vi "Delete Chan Group.vi"(8 "error in (no error)":errorcluster, 11 "Cfg Grandmaster in":refnum<class "Cfg Grandmaster.lvclass">) -> (0 "error out":errorcluster, 3 "Cfg Grandmaster out":refnum<class "Cfg Grandmaster.lvclass">)   [LabVIEW 2012, in "Configuration Grandmaster.lvlib" / "Cfg Grandmaster.lvclass"]
uses:
  Cfg Grandmaster.lvclass
  Cfg Grandmaster.lvclass/Cfg Grandmaster.ctl
  Class Chassis Cfg/ChassisCfg.lvclass
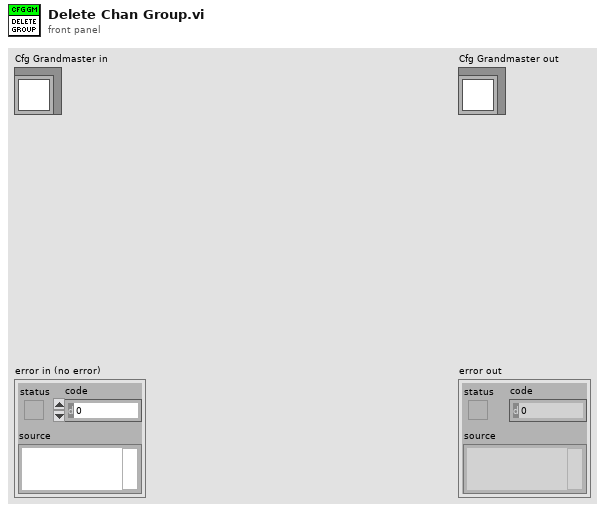
[diagram p1: front panel]
types:
  T1 = typedef "ge_Cfg wChassis.ctl" = cluster{"Chassis BOM":refnum<class "Chassis BOM.lvclass">, "Chassis Cfg":refnum<class "ChassisCfg.lvclass">, "Chassis Tasks":refnum<class "Chassis Tasks.lvclass">, "HW Error":bool, "Unsvd Chgs?":bool}
  T2 = typedef "Selected Group.ctl" = cluster{"ChanGroup":i32, "Rate Class":T3}
  T3 = typedef "TE_Designator.ctl" = enum16{"High Speed", "Low Speed"}
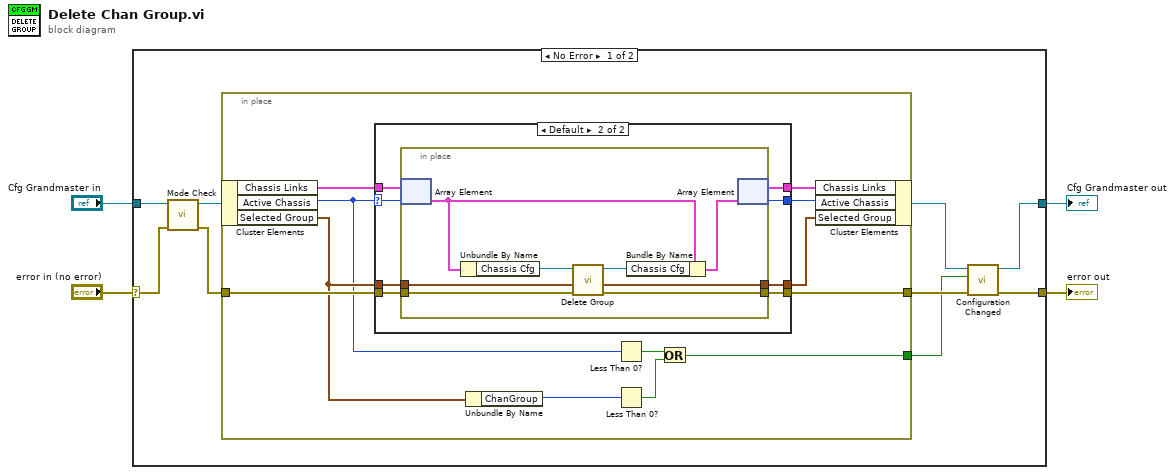
[diagram p0: block diagram]
diagram:
  n1 = case shown="No Error" "error in (no error)" {
    selector: "error in (no error)" -> [w10 w47]
    tunnel: [w8 w47] -> w3
    tunnel: [w6 w46] -> w1
    tunnel: "Cfg Grandmaster in" -> [w13 w46]
    frame No Error {
      n2 = call "Mode Check.vi"("error in (no error)"=w10, "Cfg Grandmaster in"=w13) -> ("error out"=w11:errorcluster, "Cfg Grandmaster out"=w12:refnum<class "Cfg Grandmaster.lvclass">)  [unwired: 8 in]
      n3 = in-place {
        in-place-border: w11 -> [w21]
        in-place-border: [w17] -> w9
        in-place-border: [w14] -> w5
        n4 = in-place-cluster #1(w12) -> ("Chassis Links"=w22:T1[], "Active Chassis"=w15:i32, "Selected Group"=w20:T2)
        n5 = case shown="Default" w15 {
          selector: w15 -> [w26 w32]
          tunnel: w20 -> [w27 w37]
          tunnel: w21 -> [w28 w36]
          tunnel: [w28 w35] -> w17
          tunnel: w22 -> [w29 w34]
          tunnel: [w29 w33] -> w19
          tunnel: [w26 w31] -> w18
          tunnel: [w27 w30] -> w16
          frame -1 {
          }
          frame Default {
            n6 = in-place {
              in-place-border: w37 -> [w45]
              in-place-border: w36 -> [w44]
              in-place-border: [w43] -> w35
              in-place-border: [w38] -> w30
              n7 = in-place-array #2(w34, w32) -> (w42:T1)
              n8 = Unbundle By Name(w42) -> ("Chassis Cfg"=w40:refnum<class "ChassisCfg.lvclass">)
              n9 = call "Delete Group.vi"("error in"=w44, "Selected Group"=w45, "Chassis Cfg"=w40) -> ("error out"=w43:errorcluster, "Selected Group"=w38:T2, "Chassis Cfg"=w39:refnum<class "ChassisCfg.lvclass">)  [unwired: 5 in, 1 out]
              n10 = Bundle By Name(cluster=w42, "Chassis Cfg"=w39) -> (w41:T1)
              n11 = in-place-array #2(w41) -> (w33:T1[], w31:i32)
            }
          }
        }
        n12 = Unbundle By Name(w20) -> ("ChanGroup"=w25:i32)
        n13 = Less Than 0?(x=w15) -> (x < 0?=w24:bool)
        n14 = Less Than 0?(x=w25) -> (x < 0?=w23:bool)
        n15 = Or(x=w24, y=w23) -> (x .or. y?=w14:bool)
        n16 = in-place-cluster #1("Chassis Links"=w19, "Active Chassis"=w18, "Selected Group"=w16) -> (w7:refnum<class "Cfg Grandmaster.lvclass">)
      }
      n17 = call "Configuration Changed.vi"("error in (no error)"=w9, "Canceled? (F)"=w5, "Cfg Grandmaster in"=w7) -> ("error out"=w8:errorcluster, "Cfg Grandmaster out"=w6:refnum<class "Cfg Grandmaster.lvclass">)  [unwired: 7 in]
    }
    frame Error {
    }
  }
  "error out" <- w3
  "Cfg Grandmaster out" <- w1
